vi "Finish(TCP2Foxconn).vi"(7 "Bypass查詢":bool, 8 "error in (no error)":errorcluster, 9 "Result":string, 10 "Barcode":string, 11 "TCP2Foxc":string="Driver={ODBC Driver 17 for SQL Server};Server=localhost\\SQLEXPRESS;Database=YDXB01;UID=labview;PWD=123456789") -> (0 "error out":errorcluster={"status"=TRUE, "code"=-2147217900, "source"="NI_Database_API.lvlib:Conn Execute.vi->NI_Database_API.lvlib:DB Tools Select Data.vi->Select WebCam BBOX.vi<ERR>ADO Error: 0x80040E14\r\nException occured in Microsoft OLE DB Provider for ODBC Drivers: [Microsoft][ODBC Driver 17 for SQL Server][SQL Server]接近 ',' 之處的語法不正確。 in NI_Database_API.lvlib:Conn Execute.vi->NI_Database_API.lvlib:DB Tools Select Data.vi->Select WebCam BBOX.vi"}, 2 "result":string)   [LabVIEW 2019, in "TCP2Foxconn.lvlib"]
uses:
  TCP2Foxconn.lvlib
panel:
  out "break":bool
  out "Connect?":bool
  out "times":i32
  # "True為OK"
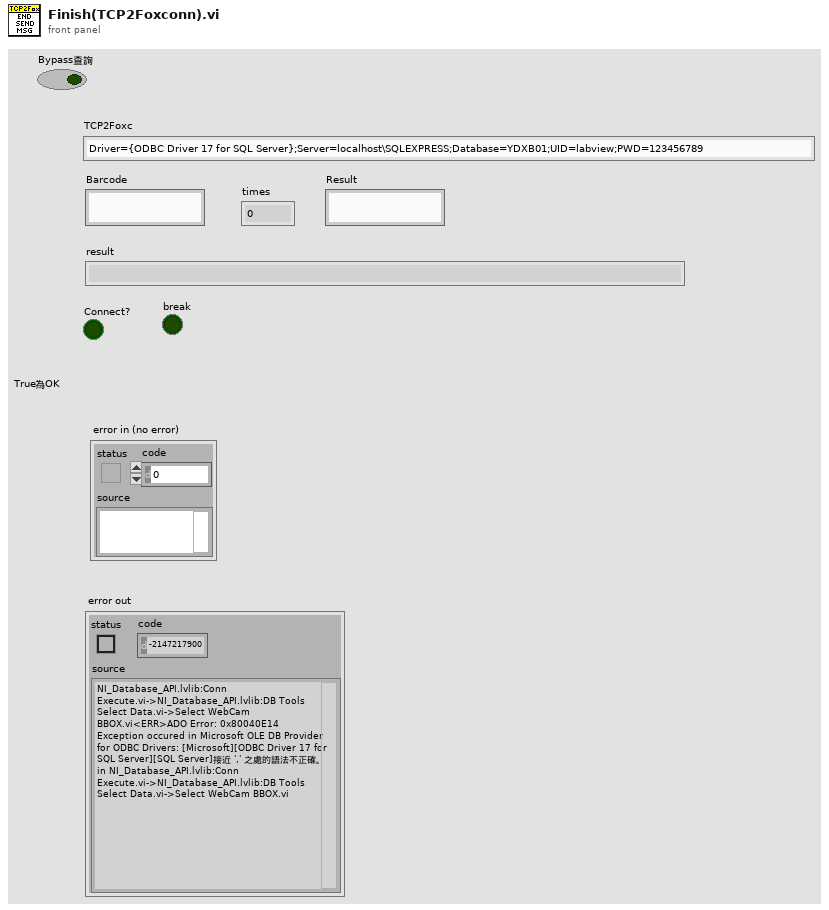
[diagram p1: front panel]
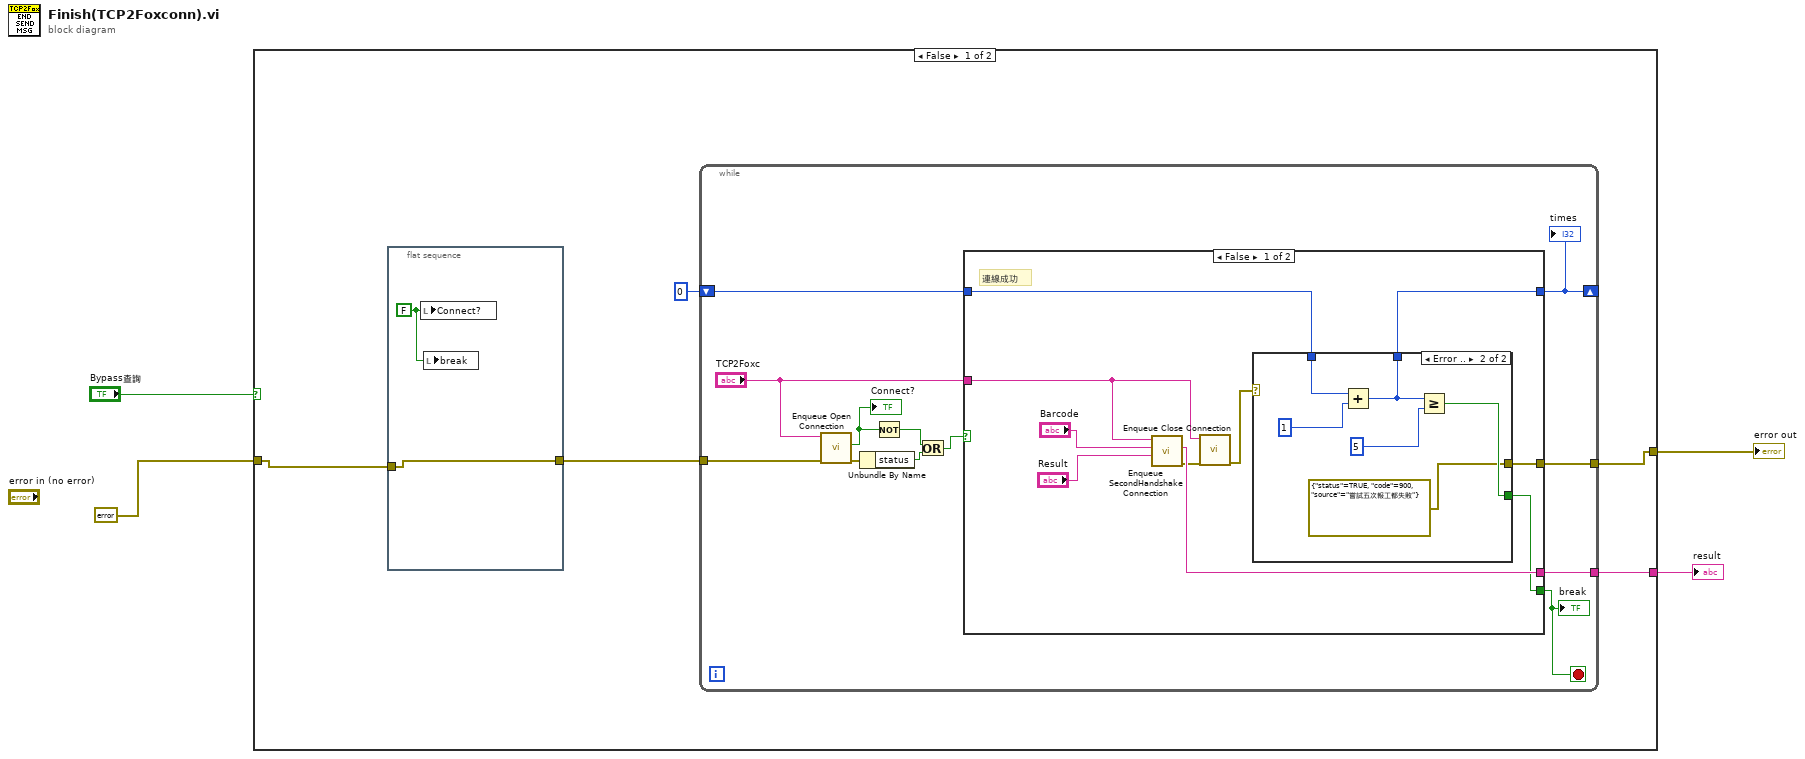
[diagram p0: block diagram]
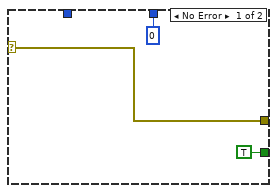
[diagram p2: hidden frame]
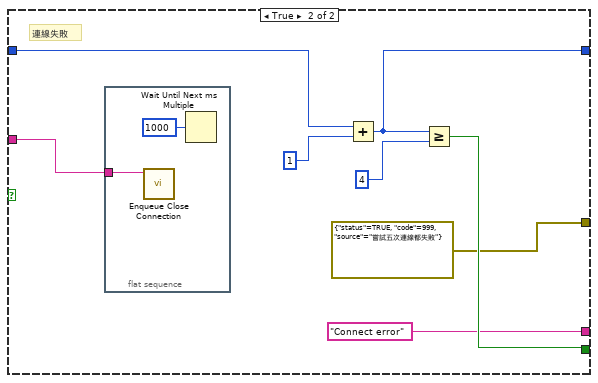
[diagram p3: hidden frame]
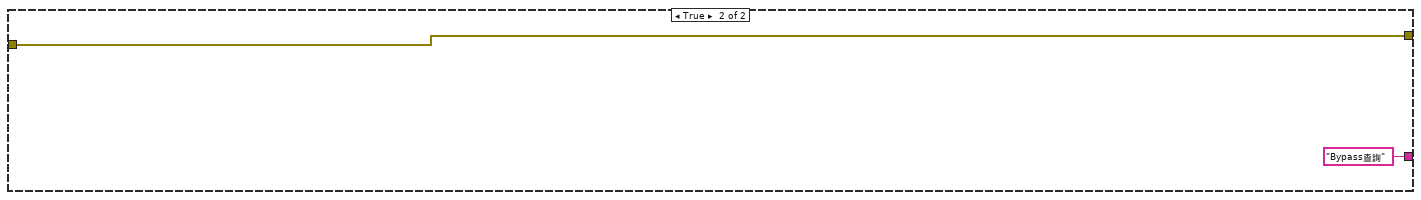
[diagram p4: hidden frame]
diagram:
  n1 = case shown="False" "Bypass查詢" {
    tunnel: [w9 "Bypass查詢"] -> w4
    tunnel: errorcluster {"status"=FALSE, "code"=0, "source"=""} ("error in (no error)") -> [w6 w53]
    tunnel: [w8 w53] -> w2
    frame False {
      n2 = flat-sequence {
        tunnel: w6 -> [w10]
        tunnel: [w10] -> w5
        frame #0 {
          w11 = FALSE ("Connect?")
          n3 = local write "Connect?"(w11) -> ()
          n4 = local write "break"(w11) -> ()
        }
      }
      n5 = while {
        tunnel: w5 -> [w23]
        tunnel: [w16] -> w9
        tunnel: [w15] -> w8
        shift-right: [w12] -> _
        shift-left: 0 -> [w14]
        stop <- w13 stop-if-true
        n6 = call "Enqueue Open Connection.vi"("Error In"=w23, "Name"="TCP2Foxc") -> ("Error Out"=w22:errorcluster, "Connect?"=w21:bool)  [unwired: 8 in]
        "Connect?" <- w21
        n7 = Unbundle By Name(w22) -> ("status"=w20:bool)
        n8 = Not(x=w21) -> (.not. x?=w19:bool)
        n9 = Or(x=w19, y=w20) -> (x .or. y?=w18:bool)
        n10 = case shown="False" w18 {
          tunnel: "TCP2Foxc" -> [w33 w44]
          tunnel: [w31 "Connect error" ("Result")] -> w16
          tunnel: [w26 errorcluster {"status"=TRUE, "code"=999, "source"="嘗試五次連線都失敗"} ("error constant")] -> w15
          tunnel: w14 -> [w25 w50]
          tunnel: [w27 w47] -> w13
          tunnel: [w24 w43] -> w12
          frame False {
            # "連線成功"
            n11 = call "Enqueue SecondHandshake Connection.vi"("Result"="Result", "Barcode"="Barcode", "Name"=w33) -> ("Error Out"=w30:errorcluster, "Result"=w31:string)  [unwired: 7 in]
            n12 = call "Enqueue Close Connection.vi"("Error In"=w30, "Name"=w33) -> ("Error Out"=w28:errorcluster)  [unwired: 9 in]
            n13 = case shown="Error .." w28 {
              selector: w28 -> [w35 _]
              tunnel: [TRUE w39] -> w27
              tunnel: [w35 errorcluster {"status"=TRUE, "code"=900, "source"="嘗試五次報工都失敗"} ("error constant")] -> w26
              tunnel: w25 -> [_ w40]
              tunnel: [0 w38] -> w24
              frame No Error {
              }
              frame Error {
                n14 = Add(x=w40, y=1) -> (x+y=w38:i32)
                n15 = Greater Or Equal?(x=w38, y=5) -> (x >= y?=w39:bool)
              }
            }
          }
          frame True {
            # "連線失敗"
            n16 = flat-sequence {
              tunnel: w44 -> [w51]
              frame #0 {
                n17 = call "Enqueue Close Connection.vi"("Name"=w51) -> ()  [unwired: 10 in, 1 out]
                n18 = Wait Until Next ms Multiple(millisecond multiple=u32 1000) -> ()  [unwired: 1 out]
              }
            }
            n19 = Add(x=w50, y=1) -> (x+y=w43:i32)
            n20 = Greater Or Equal?(x=w43, y=4) -> (x >= y?=w47:bool)
          }
        }
        "break" <- w13
        "times" <- w12
      }
    }
    frame True {
    }
  }
  "result" <- w4
  "error out" <- w2
